vi "E08_CASE.vi"() -> ()   [LabVIEW 2026]
panel:
  out "String 2":string
  out "String":string
  in  "Boolean":bool
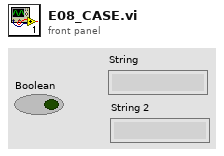
[diagram p1: front panel]
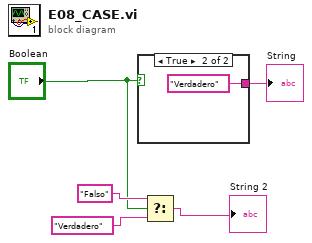
[diagram p0: block diagram]
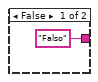
[diagram p2: hidden frame]
diagram:
  n1 = case shown="True" "Boolean" {
    tunnel: ["Falso" "Verdadero"] -> w5
    frame False {
    }
    frame True {
    }
  }
  "String" <- w5
  n2 = Select(t="Falso", s="Boolean", f="Verdadero") -> (s? t:f=→"String 2":string)
